vi "2100_Test_Set State_Measure Resistance_SH3T_Ron.vi"(0 "Semiconductor Module Context":T7, 1 "USID":T4 max=15, 2 "Publishable IDs":string[](array[string])=["State00", "State01", "State02", "State04", "State08"], 3 "R_Guardian":dbl[](array[numeric]), 5 "Script_Info":T3={"Script Name"="WalkingState", "All_Scripts"=[]}, 7 "Current  Level":dbl=0.01, 9 "Instrument_Pins":T6={"SMU_Pins"=["RF1", "RF2", "RF3", "RF4"], "HSDIO_Pins"=["CLK", "SDA"]}, 11 "Error In":errorcluster, 12 "Master_Register_Data_Array_In":T1 {"Address" format="%.0x"}, 13 "Reg_Map_and_Bit_Name":T5={"Reg_Map_Bit_Name"="", "Reg_Map"=[["Reg Addr(0x00)", "7", "6", "5", "4", "3", "2", "1", "0"], ["0", "SPARE", "RF3_SH", "RF2_SH", "RF1_SH", "SPARE", "RF3_RFC", "RF2_RFC", "RF1_RFC"], ["1", "SPARE[7:0]", "", "", "", "", "", "", ""], ["2", "VVAR_EN", "LCM_EN", "RFC_SH", "SPARE", "VARACTOR[3:0]", "", "", ""], ["3", "SW_CTRL1_VIRTUAL[7:0]", "", "", "", "", "", "", ""], ["4", "SW_CTRL1_SWAP", "SW_CTRL1_RBSHIFT[2:0]", "", "", "SW_CTRL1_VSID[3:0]", "", "", ""], ["5", "REG_00_VIRTUAL_MASK[7:0]", "", "", "", "", "", "", ""], ["6", "LOCK_STATUS[1:0]", "", "CLK_DITHER", "FUSES_BURNED", "CLK_IDAC_CAL[3:0]", "", "", ""], ["7", "SPARE[2:0]", "", "", "ODFT_TRIM[4:0]", "", "", "", ""], ["8", "SPARE[2:0]", "", "", "HV_TRIM[4:0]", "", "", "", ""], ["9", "TEST_MUX[2:0]", "", "", "SPARE[1:0]", "", "MEMS_BG_TC[1:0]", "", "MEMSCP_RCM"], ["A", "CP_BOOST_OVRD_EN", "SPARE[2:0]", "", "", "PS_OFF_TIMER[1:0]", "", "PS_ON_TIMER[1:0]", ""], ["0", "", "", "", "", "", "", "", ""], ["D", "Reserved[1:0]", "", "WD_HI_EVENT_CNT[5:0]", "", "", "", "", ""], ["E", "VERSION_ID[7:0]", "", "", "", "", "", "", ""], ["F", "Reserved", "COUNT_200_LSB[6:0]", "", "", "", "", "", ""], ["10", "CLK_DIV2_EN", "Spare", "ODFT_EN", "HV_HYST[4:0]", "", "", "", ""], ["0", "", "", "", "", "", "", "", ""], ["12", "SHORT_FUSE", "FUSE_BURN", "STROBE_EN", "VIO_OK", "RTH[1:0]", "", "FUSE_LOAD_MAN_EN", "FUSE_LOAD"], ["13", "RR_ACK_EN", "Reserved", "ACK_POSITION[1:0]", "", "SuBUS_DRIVE_STRENGTH[3:0]", "", "", ""], ["14", "TM_IO_EN", "TM_IO_SEL", "SuBUS_OVS[1:0]", "", "Reserved[3:0]", "", "", ""], ["15", "Reserved[4:0]", "", "", "", "", "SuBUS_VERSION_PRESENT", "SuBUS_VOLTAGE", "SuBUS_FLAVOR_DEF"], ["16", "PROG_STROBE1_DUR[7:0]", "", "", "", "", "", "", ""], ["17", "PROG_STROBE0_DUR[7:0]", "", "", "", "", "", "", ""], ["18", "Reserved[2:0]", "", "", "EFUSE_SINGLE_ADDR_SEL[4:0]", "", "", "", ""], ["19", "POLL_ADR[4:0]", "", "", "", "", "POLL_BC[2:0]", "", ""], ["1A", "SOFTWARE_RESET", "Reserved[6:0]", "", "", "", "", "", ""], ["1B", "Reserved[7:0]", "", "", "", "", "", "", ""], ["1C", "PWR_MODE_1", "PWR_MODE_0", "TRIGGER_MASK[2:0]", "", "", "TRIGGER[2:0]", "", ""], ["1D", "PRODUCT_ID[7:0]", "", "", "", "", "", "", ""], ["1E", "MANUFACTURER_ID_LSB[7:0]", "", "", "", "", "", "", ""], ["1F", "MANUFACTURER_ID_MSB[3:0]", "", "", "", "USID[3:0]", "", "", ""]]}) -> (6 "Master_Register_Data_Array_Out":T1 {"Address" format="%.0x"}, 15 "Error Out":errorcluster)   [LabVIEW 2013]
uses:
  Controls/USID.ctl
  <vilib>/NI_TestStand_SemiconductorModule/NI_TestStand_Semiconductor_Module.lvlibp/PinMap/General/SemiconductorModuleContext.ctl
  Controls/Master_Reg_Data_Array.ctl
  Controls/Reg_Address_Data.ctl
  <vilib>/NI_TestStand_SemiconductorModule/NI_TestStand_Semiconductor_Module.lvlibp/PinMap/General/Publish/PublishDataDoubleFunctionalTest.vi
  <vilib>/NI_TestStand_SemiconductorModule/NI_TestStand_Semiconductor_Module.lvlibp
panel:
  out "Publishable IDs 2":string[](array[string])=["State00", "State01", "State02", "State04", "State08"]
  out "Logged_Data":dbl[](array[numeric]) format="%#_6p"
  out "R_Measurements":dbl[](array[numeric]) format="%#_6p"
  in  "Tab Control":enum32{"Test Info", "Instrument Settings"}(tab)
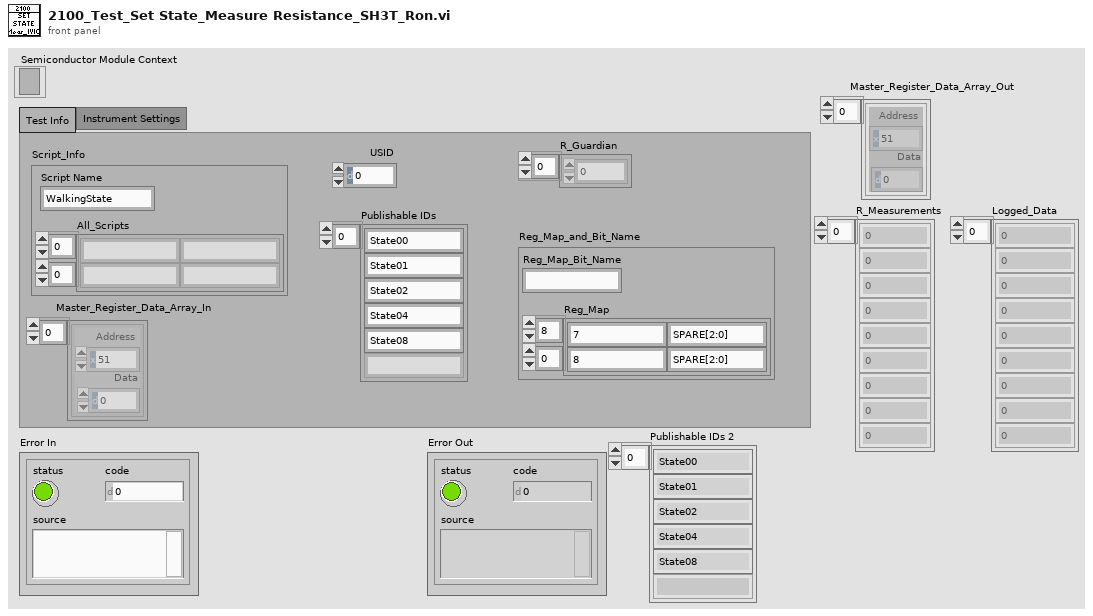
[diagram p1: front panel]
types:
  T1 = typedef "Master_Reg_Data_Array.ctl" = T2[]
  T2 = typedef "Reg_Address_Data.ctl" = cluster{"Address":u8, "Data":u8}
  T3 = cluster{"Script Name":string, "All_Scripts":string[][]}
  T4 = typedef "USID.ctl" = u8
  T5 = cluster{"Reg_Map_Bit_Name":string, "Reg_Map":string[][]}
  T6 = cluster{"SMU_Pins":string[], "HSDIO_Pins":string[]}
  T7 = typedef "NI_TestStand_Semiconductor_Module.lvlibp/SemiconductorModuleContext.ctl" = refnum<k7>
  T8 = typedef "Script Functions_Array.ctl" = enum16{"Reg_Write", "Bit_Write", "Delay", "Read", "Measure"}[]
  T9 = enum16{"Reg_Write", "Bit_Write", "Delay", "Read", "Measure"}
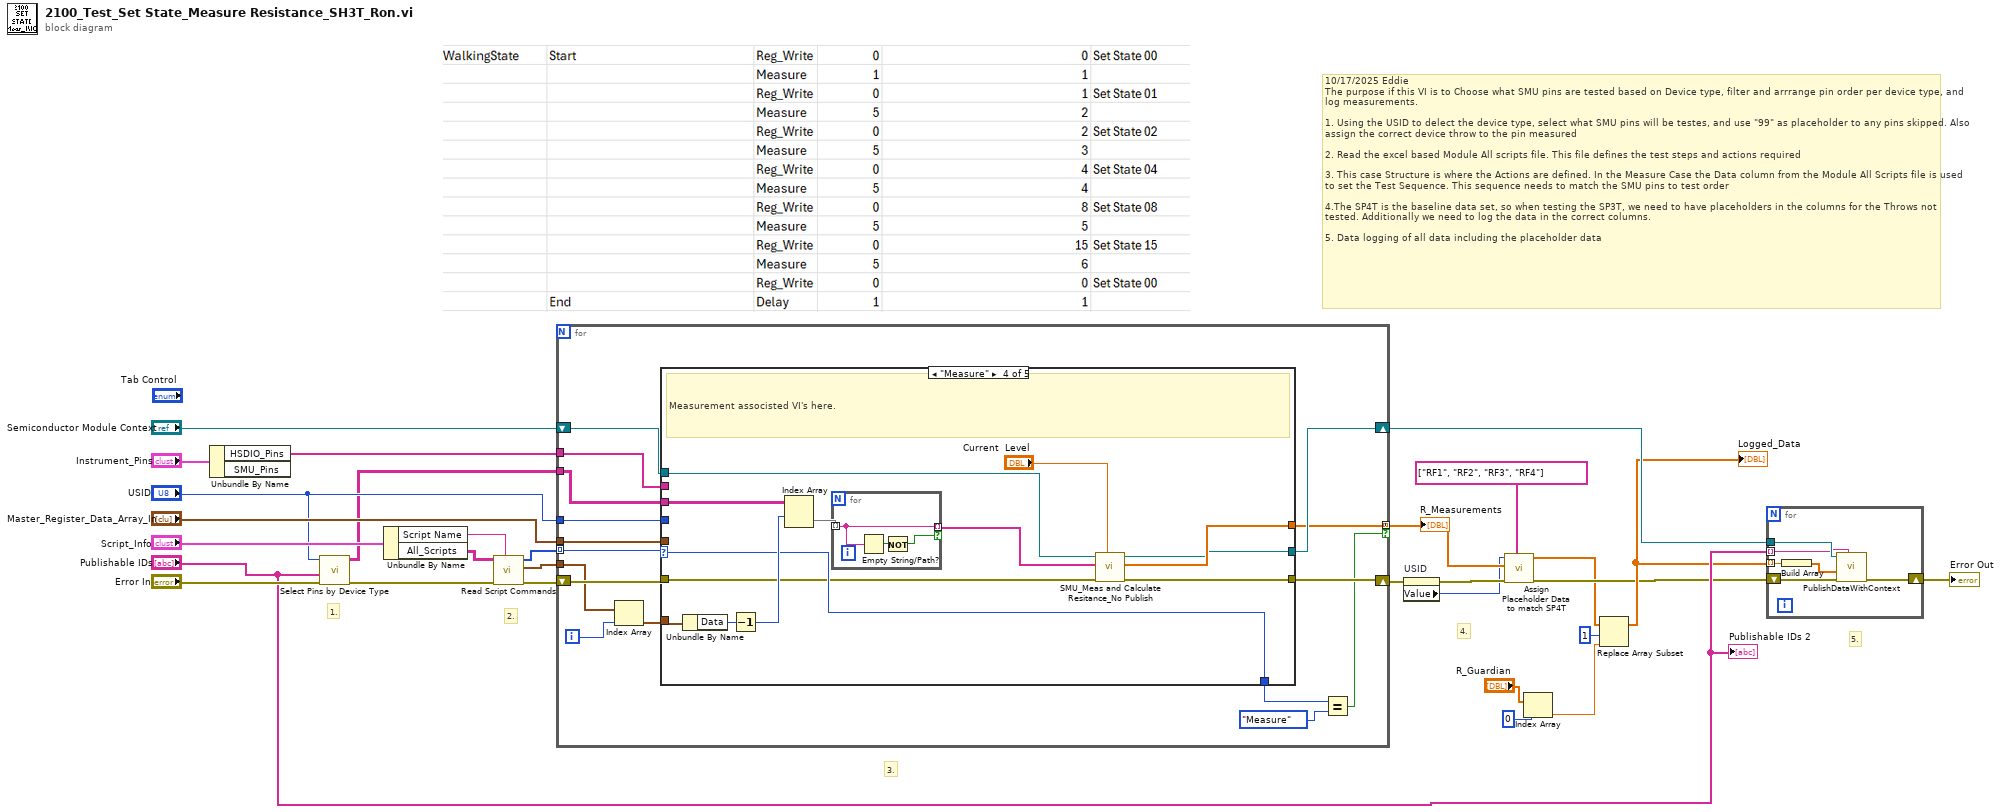
[diagram p0: block diagram]
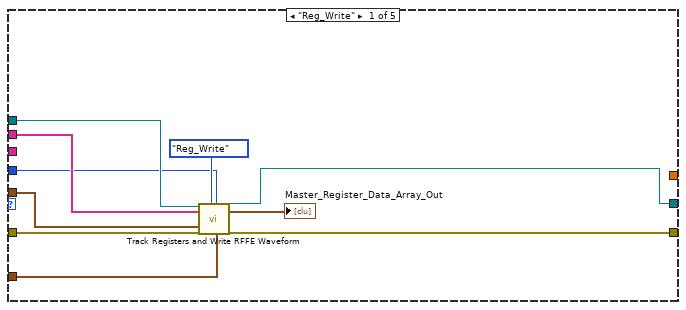
[diagram p2: hidden frame]
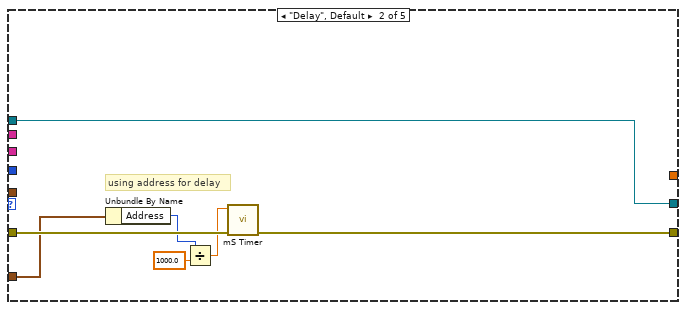
[diagram p3: hidden frame]
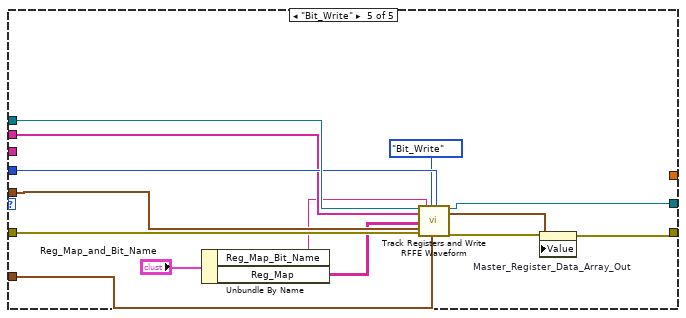
[diagram p5: hidden frame]
diagram:
  # "10/17/2025 Eddie \nThe purpose if this VI is to Choose what SMU pins are tested based on Device type, filter and arrrange pin order per device type, and log measurements.\n\n1. Using the USID to delect the device type, select what SMU pins will be testes, and use \"99\" as placeholder to any pins skipped. Also assign the correct device throw to the pin measured\n\n2. Read the excel based Module All scripts file. This file defines the test steps and actions required\n\n3. This case Structure is where the Actions are defined. In the Measure Case the Data column from the Module All Scripts file is used to set the Test Sequence. This sequence needs to match the SMU pins to test order\n\n4.The SP4T is the baseline data set, so when testing the SP3T, we need to have placeholders in the columns for the Throws not tested. Additionally we need to log the data in the correct columns.\n\n5. Data logging of all data including the placeholder data"
  # "5."
  # "4."
  # "3."
  # "2."
  # "1."
  n1 = Unbundle By Name("Instrument_Pins") -> ("HSDIO_Pins"=w23:string[])  [unwired: 1 out]
  n2 = call "Select Pins by Device Type.vi"("error in (no error)"="Error In", "Publishable IDs"="Publishable IDs", "USID"="USID") -> ("error out"=w18:errorcluster, "Pins to Test"=w16:string[][])  [unwired: 7 in]
  n3 = Unbundle By Name("Script_Info") -> ("Script Name"=w20:string, "All_Scripts"=w21:string[][])
  n4 = call "Read Script Commands.vi"("Test Name"=w20, "Error In"=w18, "All_Scripts"=w21) -> ("Error Out"=w27:errorcluster, "Script_Data"=w28:T2[], "Script_Functions"=w29:T8)  [unwired: 5 in, 1 out]
  n5 = for {
    tunnel: "USID" -> [w39]
    tunnel: w29 -> [w38] mode=indexing
    tunnel: w28 -> [w42]
    tunnel: w23 -> [w43]
    shift-right: [w36] -> w3
    shift-left: w27 -> [w45]
    tunnel: "Master_Register_Data_Array_In" -> [w40]
    tunnel: w16 -> [w35]
    shift-right: [w34] -> w14
    shift-left: "Semiconductor Module Context" -> [w44]
    tunnel: [w33] -> w6 mode=concatenating if=w30
    i -> [w37]
    n6 = Index Array(array=w42, index=w37) -> (element=w41:T2)
    n7 = case shown="\"Measure\"" w38 {
      selector: w38 -> [_ _ _ w72 _]
      tunnel: w41 -> [w50 w61 _ w77 w81]
      tunnel: w45 -> [w55 w62 w64 w71 w94]
      tunnel: w39 -> [w47 _ _ _ w88]
      tunnel: w44 -> [w53 w56 w63 w69 w89]
      tunnel: w43 -> [w52 _ _ _ w86]
      tunnel: [w54 w60 w64 w70 w92] -> w36
      tunnel: w40 -> [w49 _ _ _ w85]
      tunnel: w35 -> [_ _ _ w76 _]
      tunnel: [w46 w56 w63 w65 w90] -> w34
      tunnel: [_ _ _ w66 _] -> w33
      tunnel: [_ _ _ w72 _] -> w32
      frame "Reg_Write" {
        n8 = call "Track Registers and Write RFFE Waveform.vi"("Semiconductor Module Context"=w53, "Pins"=w52, "Master_Register_Data_Array_In"=w49, "Error In"=w55, "Script_Functions"=enum16{"Reg_Write", "Bit_Write"}."Reg_Write", "USID"=w47, "Reg_Address_Data"=w50) -> ("Semiconductor Module Context Out"=w46:T7, "Master_Register_Data_Array_Out"=→"Master_Register_Data_Array_Out":T1, "Error Out"=w54:errorcluster)  [unwired: 10 in]
      }
      frame "Delay", Default {
        # "using address for delay"
        n9 = Unbundle By Name(w61) -> ("Address"=w58:u8)
        n10 = Divide(x=w58, y=1000.0) -> (x/y=w57:dbl)
        n11 = call "mS Timer.vi"("Error In"=w62, "Delay(S)"=w57) -> ("Error Out"=w60:errorcluster)  [unwired: 9 in]
      }
      frame "Read" {
        # "Future Dev Code"
      }
      frame "Measure" {
        # "Measurement associsted VI's here."
        n12 = Unbundle By Name(w77) -> ("Data"=w74:u8)
        n13 = Decrement(x=w74) -> (x-1=w73:u8)
        n14 = Index Array(array=w76, index (row)=w73) -> (element=w75:string[])  [unwired: 1 in]
        n15 = for {
          tunnel: w75 -> [w80] mode=indexing
          tunnel: [w80] -> w67 mode=indexing if=w78
          n16 = Empty String/Path?(string/path=w80) -> (empty?=w79:bool)
          n17 = Not(x=w79) -> (.not. x?=w78:bool)
        }
        n18 = call "SMU_Meas and Calculate Resitance_No Publish.vi"("Current  Level"="Current  Level", "error in (no error)"=w71, "Pins"=w67, "Semiconductor Module Context"=w69) -> ("error Out"=w70:errorcluster, "R Array"=w66:dbl[], "Semiconductor Module Context Out"=w65:T7)  [unwired: 5 in]
      }
      frame "Bit_Write" {
        n19 = Unbundle By Name("Reg_Map_and_Bit_Name") -> ("Reg_Map_Bit_Name"=w83:string, "Reg_Map"=w82:string[][])
        n20 = call "Track Registers and Write RFFE Waveform.vi"("Semiconductor Module Context"=w89, "Pins"=w86, "Reg_Map"=w82, "Master_Register_Data_Array_In"=w85, "Error In"=w94, "Reg_Map_Bit_Name"=w83, "Script_Functions"=enum16{"Reg_Write", "Bit_Write"}."Bit_Write", "USID"=w88, "Reg_Address_Data"=w81) -> ("Semiconductor Module Context Out"=w90:T7, "Master_Register_Data_Array_Out"=w91:T1, "Error Out"=w93:errorcluster)  [unwired: 8 in]
        n21 = property on="Master_Register_Data_Array_Out" class="Arr (strict)"(error in=w93, "Value"=w91) -> (error out=w92:errorcluster)  [unwired: 1 in, 1 out]
      }
    }
    n22 = Equal?(x=w32, y=T9."Measure" ("Enum")) -> (x = y?=w30:bool)
  }
  "R_Measurements" <- w6
  n23 = property on="USID" class="DigNum (strict)"(error in=w3) -> (error out=w2:errorcluster, "Value"=w1:T4)  [unwired: 1 in, 1 out]
  n24 = call "Assign Placeholder Data to match SP4T.vi"("SP4T_Pins"=string[] ["RF1", "RF2", "RF3", "RF4"], "error in (no error)"=w2, "Individual_R_Meas"=w6, "USID"=w1) -> ("error out"=w8:errorcluster, "Placeholder_w_Data"=w5:dbl[])  [unwired: 6 in]
  n25 = Index Array(array="R_Guardian", index=0) -> (element=w9:dbl)
  n26 = Replace Array Subset(array=w5, new element=w9, index=1) -> (w10:dbl[])
  "Logged_Data" <- w10
  n27 = for {
    shift-right: [w100] -> w15
    shift-left: w8 -> [w99]
    tunnel: w14 -> [w98]
    tunnel: w10 -> [w97] mode=indexing
    tunnel: "Publishable IDs" -> [w95] mode=indexing
    n28 = Build Array(w97) -> (w96:dbl[])
    n29 = call-poly <vilib>:"PublishDataWithContext.vi"("Published Data Id"=w95, "error in (no error)"=w99, "Data In"=w96, "Semiconductor Module Context"=w98) -> ("error out"=w100:errorcluster)  [unwired: 6 in, 1 out]
  }
  "Error Out" <- w15
  "Publishable IDs 2" <- "Publishable IDs"
